vi "Initialize Front Panel.vi"(8 "error in (no error)":errorcluster, 11 "File Explorer in":refnum<class "File Explorer.lvclass">) -> (0 "error out":errorcluster, 3 "File Explorer out":refnum<class "File Explorer.lvclass">)   [LabVIEW 2017, in "File Explorer.lvlib" / "File Explorer.lvclass"]
doc: "<License>\nCopyright © 2017 Composed Systems, LLC | All rights reserved\nwww.composed.io\n\nAuthor: Ethan Stern <ethan.stern@composed.io>\n\nThis software is provided \"AS IS\" WITHOUT WARRANTIES, either express or implied, AND IS FOR EDUCATIONAL PURPOSES ONLY.\n</License>"
uses:
  <vilib>/gpm_packages/@cs/file-explorer-extension/Source/File Explorer/File Explorer/File Explorer.lvclass
  <vilib>/gpm_packages/@cs/mva-viewable/Source/IViewable/IViewable/IViewable.lvclass
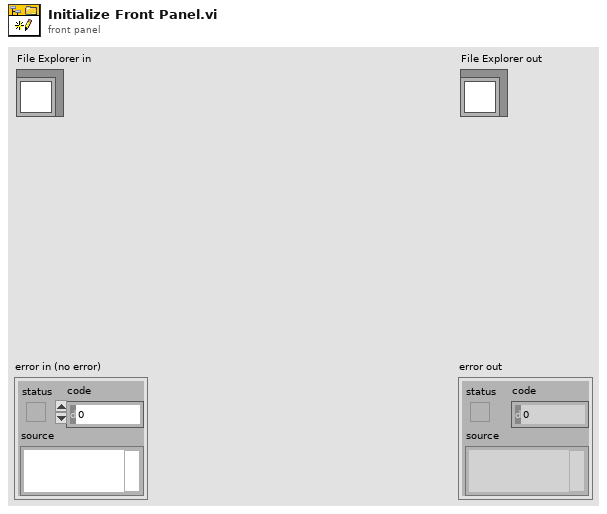
[diagram p1: front panel]
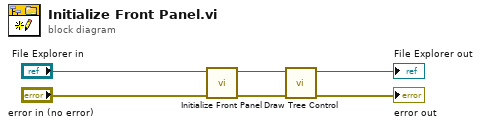
[diagram p0: block diagram]
diagram:
  n1 = call-parent "Initialize Front Panel.vi"("error in (no error)"="error in (no error)", "IViewable in"="File Explorer in") -> ("error out"=w2:errorcluster, "IViewable out"=w4:refnum<class "File Explorer.lvclass">)  [unwired: 8 in]
  n2 = call <vilib>:"Draw Tree Control.vi"("error in (no error)"=w2, "File Explorer in"=w4) -> ("error out"=→"error out":errorcluster, "File Explorer out"=→"File Explorer out":refnum<class "File Explorer.lvclass">)  [unwired: 8 in]
